vi "Write DAQ Rack Data.vi"(8 "Cal Unit":T2, 9 "Channel to Cal":T1, 10 "Verify Table":string[][](array[string]), 11 "Cal Path":path) -> ()   [LabVIEW 2013]
uses:
  Type Defs/Units Type Def (DAQ Rack).ctl
  Type Defs/Channel Type Def (RIO).ctl
  Type Defs/Excel Driver Operator Type Def.ctl
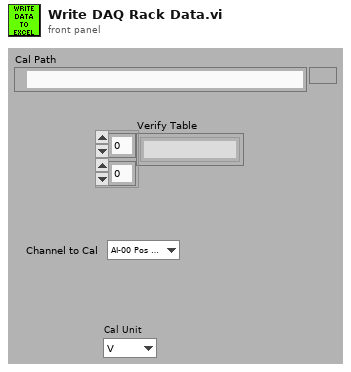
[diagram p1: front panel]
types:
  T1 = typedef "Channel Type Def (RIO).ctl" = enum16{"AI-00 Pos 1 Pump Current", "AI-01 Pos 2 Pump Current", "AI-02 Pos 3 Pump Current", "AI-03 Pos 4 Pump Current", "AI-04 Pos 5 Pump Current", "AI-05 Pos 6 Pump Current", "AI-06 Pos 1 Speed", "AI-07 Pos 2 speed", "AI-08 Pos 3 Speed", "AI-09 Pos 4 Speed", "AI-10 Pos 5 Speed", "AI-11 Pos 6 Speed", "AI-12 Pos 1 Controller Current", "AI-13 Pos 2 Controller Current", "AI-14 Pos 3 Controller Current", "AI-15 Pos 4 Controller Current", "AI-16 Pos 5 Controller Current", "AI-17 Pos 6 Controller Current", "AI-18 Spare", "AI-19 Tank 1 Temperature", "AI-20 Tank 2 Temperature", "AI-21 Power Supply Voltage", "AI-22 Pos 1 Pressure", "AI-23 Pos 2 Pressure", "AI-24 Pos 3 Pressure", "AI-25 Pos 4 Pressure", "AI-26 Pos 5 Pressure", "AI-27 Pos 6 Pressure", "AI-28 Pos 1 Flow", "AI-29 Pos 2 Flow", "AI-30 Pos 3 Flow", "AI-31 Pos 4 Flow", "AI-32 Pos 5 Flow", "AI-33 Pos 6 Flow", "AI-34 Spare", "AI-35 Spare", "AI-36 Spare", "AI-37 Spare"}
  T2 = typedef "Units Type Def (DAQ Rack).ctl" = enum16{"V", "mA", "A", "Hz", "deg C"}
  T3 = typedef "Excel Driver Operator Type Def.ctl" = enum16{"Open", "Close", "Search for String", "GetUsedRange", "Read Range", "Read Cell", "Set Range", "Set Cell"}
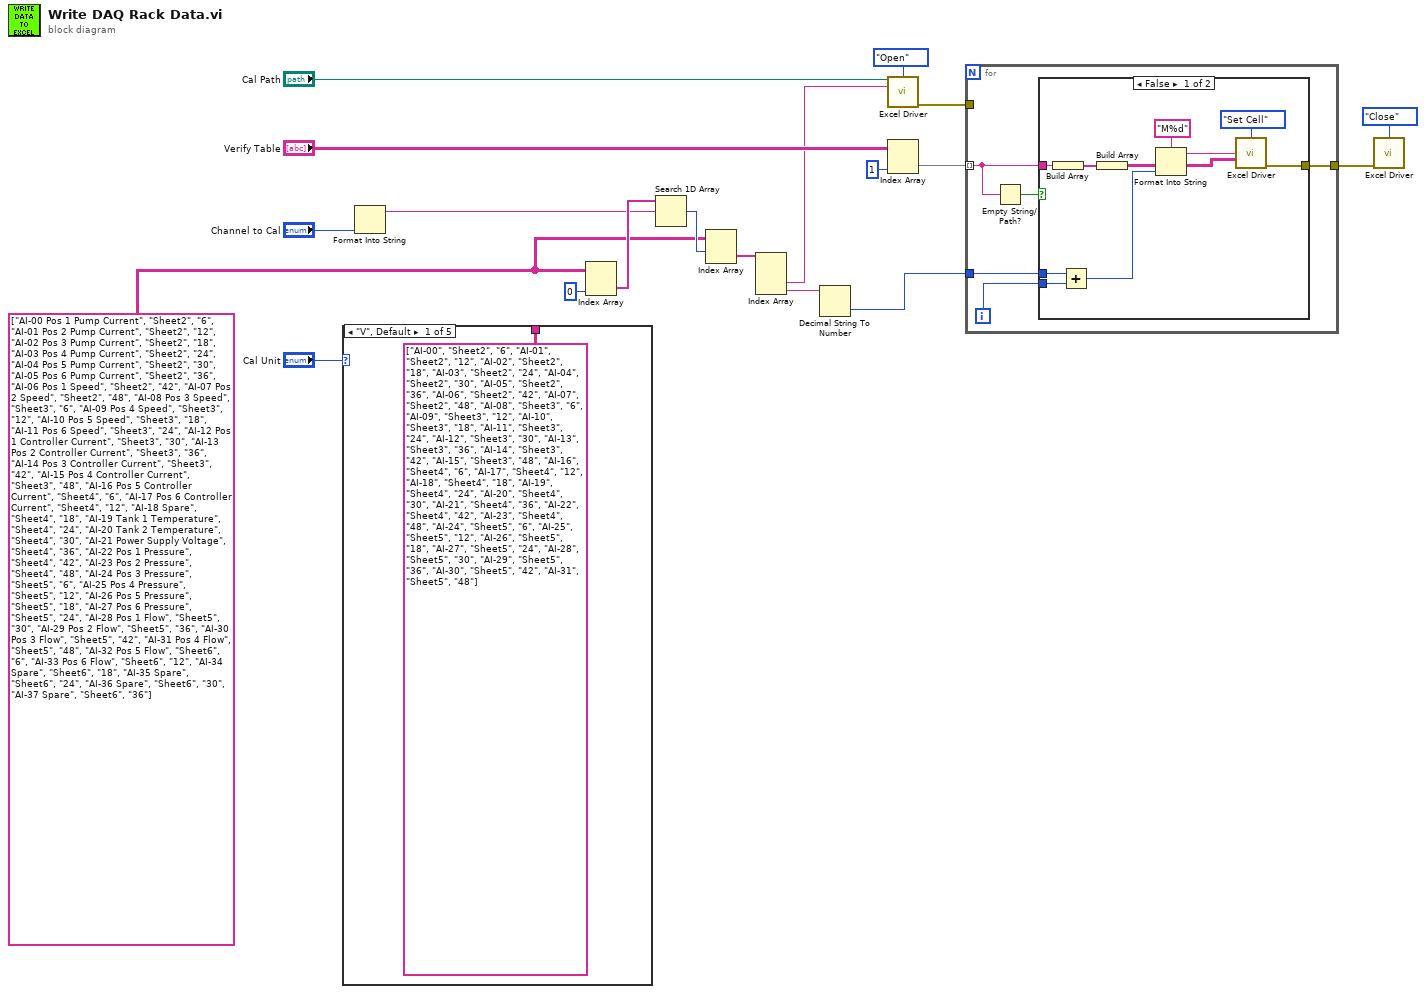
[diagram p0: block diagram]
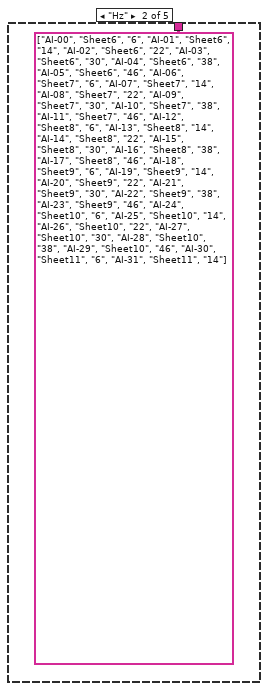
[diagram p2: hidden frame]
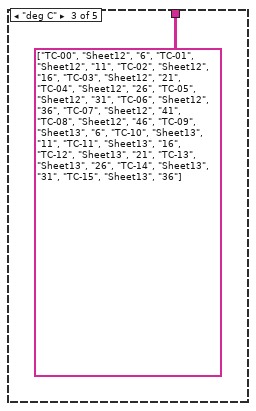
[diagram p3: hidden frame]
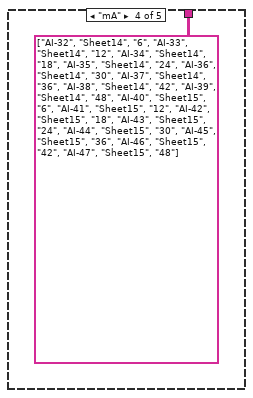
[diagram p4: hidden frame]
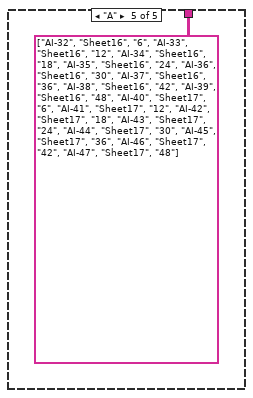
[diagram p5: hidden frame]
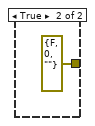
[diagram p6: hidden frame]
diagram:
  w1 = string[][] [["AI-00 Pos 1 Pump Current", "Sheet2", "6"], ["AI-01 Pos 2 Pump Current", "Sheet2", "12"], ["AI-02 Pos 3 Pump Current", "Sheet2", "18"], ["AI-03 Pos 4 Pump Current", "Sheet2", "24"], ["AI-04 Pos 5 Pump Current", "Sheet2", "30"], ["AI-05 Pos 6 Pump Current", "Sheet2", "36"], ["AI-06 Pos 1 Speed", "Sheet2", "42"], ["AI-07 Pos 2 Speed", "Sheet2", "48"], ["AI-08 Pos 3 Speed", "Sheet3", "6"], ["AI-09 Pos 4 Speed", "Sheet3", "12"], ["AI-10 Pos 5 Speed", "Sheet3", "18"], ["AI-11 Pos 6 Speed", "Sheet3", "24"], ["AI-12 Pos 1 Controller Current", "Sheet3", "30"], ["AI-13 Pos 2 Controller Current", "Sheet3", "36"], ["AI-14 Pos 3 Controller Current", "Sheet3", "42"], ["AI-15 Pos 4 Controller Current", "Sheet3", "48"], ["AI-16 Pos 5 Controller Current", "Sheet4", "6"], ["AI-17 Pos 6 Controller Current", "Sheet4", "12"], ["AI-18 Spare", "Sheet4", "18"], ["AI-19 Tank 1 Temperature", "Sheet4", "24"], ["AI-20 Tank 2 Temperature", "Sheet4", "30"], ["AI-21 Power Supply Voltage", "Sheet4", "36"], ["AI-22 Pos 1 Pressure", "Sheet4", "42"], ["AI-23 Pos 2 Pressure", "Sheet4", "48"], ["AI-24 Pos 3 Pressure", "Sheet5", "6"], ["AI-25 Pos 4 Pressure", "Sheet5", "12"], ["AI-26 Pos 5 Pressure", "Sheet5", "18"], ["AI-27 Pos 6 Pressure", "Sheet5", "24"], ["AI-28 Pos 1 Flow", "Sheet5", "30"], ["AI-29 Pos 2 Flow", "Sheet5", "36"], ["AI-30 Pos 3 Flow", "Sheet5", "42"], ["AI-31 Pos 4 Flow", "Sheet5", "48"], ["AI-32 Pos 5 Flow", "Sheet6", "6"], ["AI-33 Pos 6 Flow", "Sheet6", "12"], ["AI-34 Spare", "Sheet6", "18"], ["AI-35 Spare", "Sheet6", "24"], ["AI-36 Spare", "Sheet6", "30"], ["AI-37 Spare", "Sheet6", "36"]] ("deleted portion")
  n1 = case shown="\"V\", Default" "Cal Unit" {
    tunnel: [string[][] [["AI-00", "Sheet2", "6"], ["AI-01", "Sheet2", "12"], ["AI-02", "Sheet2", "18"], ["AI-03", "Sheet2", "24"], ["AI-04", "Sheet2", "30"], ["AI-05", "Sheet2", "36"], ["AI-06", "Sheet2", "42"], ["AI-07", "Sheet2", "48"], ["AI-08", "Sheet3", "6"], ["AI-09", "Sheet3", "12"], ["AI-10", "Sheet3", "18"], ["AI-11", "Sheet3", "24"], ["AI-12", "Sheet3", "30"], ["AI-13", "Sheet3", "36"], ["AI-14", "Sheet3", "42"], ["AI-15", "Sheet3", "48"], ["AI-16", "Sheet4", "6"], ["AI-17", "Sheet4", "12"], ["AI-18", "Sheet4", "18"], ["AI-19", "Sheet4", "24"], ["AI-20", "Sheet4", "30"], ["AI-21", "Sheet4", "36"], ["AI-22", "Sheet4", "42"], ["AI-23", "Sheet4", "48"], ["AI-24", "Sheet5", "6"], ["AI-25", "Sheet5", "12"], ["AI-26", "Sheet5", "18"], ["AI-27", "Sheet5", "24"], ["AI-28", "Sheet5", "30"], ["AI-29", "Sheet5", "36"], ["AI-30", "Sheet5", "42"], ["AI-31", "Sheet5", "48"]] ("deleted portion") string[][] [["AI-00", "Sheet6", "6"], ["AI-01", "Sheet6", "14"], ["AI-02", "Sheet6", "22"], ["AI-03", "Sheet6", "30"], ["AI-04", "Sheet6", "38"], ["AI-05", "Sheet6", "46"], ["AI-06", "Sheet7", "6"], ["AI-07", "Sheet7", "14"], ["AI-08", "Sheet7", "22"], ["AI-09", "Sheet7", "30"], ["AI-10", "Sheet7", "38"], ["AI-11", "Sheet7", "46"], ["AI-12", "Sheet8", "6"], ["AI-13", "Sheet8", "14"], ["AI-14", "Sheet8", "22"], ["AI-15", "Sheet8", "30"], ["AI-16", "Sheet8", "38"], ["AI-17", "Sheet8", "46"], ["AI-18", "Sheet9", "6"], ["AI-19", "Sheet9", "14"], ["AI-20", "Sheet9", "22"], ["AI-21", "Sheet9", "30"], ["AI-22", "Sheet9", "38"], ["AI-23", "Sheet9", "46"], ["AI-24", "Sheet10", "6"], ["AI-25", "Sheet10", "14"], ["AI-26", "Sheet10", "22"], ["AI-27", "Sheet10", "30"], ["AI-28", "Sheet10", "38"], ["AI-29", "Sheet10", "46"], ["AI-30", "Sheet11", "6"], ["AI-31", "Sheet11", "14"]] ("deleted portion") string[][] [["TC-00", "Sheet12", "6"], ["TC-01", "Sheet12", "11"], ["TC-02", "Sheet12", "16"], ["TC-03", "Sheet12", "21"], ["TC-04", "Sheet12", "26"], ["TC-05", "Sheet12", "31"], ["TC-06", "Sheet12", "36"], ["TC-07", "Sheet12", "41"], ["TC-08", "Sheet12", "46"], ["TC-09", "Sheet13", "6"], ["TC-10", "Sheet13", "11"], ["TC-11", "Sheet13", "16"], ["TC-12", "Sheet13", "21"], ["TC-13", "Sheet13", "26"], ["TC-14", "Sheet13", "31"], ["TC-15", "Sheet13", "36"]] ("array w/ subset deleted") string[][] [["AI-32", "Sheet14", "6"], ["AI-33", "Sheet14", "12"], ["AI-34", "Sheet14", "18"], ["AI-35", "Sheet14", "24"], ["AI-36", "Sheet14", "30"], ["AI-37", "Sheet14", "36"], ["AI-38", "Sheet14", "42"], ["AI-39", "Sheet14", "48"], ["AI-40", "Sheet15", "6"], ["AI-41", "Sheet15", "12"], ["AI-42", "Sheet15", "18"], ["AI-43", "Sheet15", "24"], ["AI-44", "Sheet15", "30"], ["AI-45", "Sheet15", "36"], ["AI-46", "Sheet15", "42"], ["AI-47", "Sheet15", "48"]] ("deleted portion") string[][] [["AI-32", "Sheet16", "6"], ["AI-33", "Sheet16", "12"], ["AI-34", "Sheet16", "18"], ["AI-35", "Sheet16", "24"], ["AI-36", "Sheet16", "30"], ["AI-37", "Sheet16", "36"], ["AI-38", "Sheet16", "42"], ["AI-39", "Sheet16", "48"], ["AI-40", "Sheet17", "6"], ["AI-41", "Sheet17", "12"], ["AI-42", "Sheet17", "18"], ["AI-43", "Sheet17", "24"], ["AI-44", "Sheet17", "30"], ["AI-45", "Sheet17", "36"], ["AI-46", "Sheet17", "42"], ["AI-47", "Sheet17", "48"]] ("deleted portion")] -> _
    frame "V", Default {
    }
    frame "Hz" {
    }
    frame "deg C" {
    }
    frame "mA" {
    }
    frame "A" {
    }
  }
  n2 = Format Into String("Channel to Cal") -> (resulting string=w3:string)  [unwired: 3 in, 1 out]
  n3 = Index Array(array=w1, index (col)=0 ("disabled index (col)")) -> (element=w10:string[])  [unwired: 1 in]
  n4 = Search 1D Array(1D array=w10, element=w3) -> (index of element=w9:i32)  [unwired: 1 in]
  n5 = Index Array(array=w1, index (row)=w9) -> (element=w8:string[])  [unwired: 1 in]
  n6 = Index Array(array=w8) -> (element #2=w7:string, element #3=w6:string)  [unwired: 3 in, 1 out]
  n7 = Decimal String To Number(string=w6) -> (number=w5:i32)  [unwired: 2 in, 1 out]
  n8 = call "Excel Driver.vi"("Filename of Workbook"="Cal Path", "Operator"=Excel_Driver_Operator_Type_Def."Open", "WorkSheet Name"=w7) -> ("error out"=w15:errorcluster)  [unwired: 10 in, 2 out]
  n9 = Index Array(array="Verify Table", index (col)=1 ("disabled index (col)")) -> (element=w16:string[])  [unwired: 1 in]
  n10 = for {
    tunnel: w16 -> [w26] mode=indexing
    tunnel: w5 -> [w29]
    tunnel: w15 -> [_]
    tunnel: [w28] -> w13
    i -> [w27]
    n11 = Empty String/Path?(string/path=w26) -> (empty?=w25:bool)
    n12 = case shown="False" w25 {
      tunnel: w26 -> [w38 _]
      tunnel: w29 -> [w32 _]
      tunnel: [w31 errorcluster {"status"=FALSE, "code"=0, "source"=""} ("error out")] -> w28
      tunnel: w27 -> [w30 _]
      frame False {
        n13 = Build Array(w38) -> (w37:string[])
        n14 = Add(x=w32, y=w30) -> (x+y=w33:i32)
        n15 = Build Array(w37) -> (w36:string[][])
        n16 = Format Into String(format string="M%d", w33) -> (resulting string=w34:string)  [unwired: 2 in, 1 out]
        n17 = call "Excel Driver.vi"("Operator"=Excel_Driver_Operator_Type_Def."Set Cell", "Range String\n(Or Search String)"=w34, "Cell Values INPUT"=w36) -> ("error out"=w31:errorcluster)  [unwired: 10 in, 2 out]
      }
      frame True {
      }
    }
  }
  n18 = call "Excel Driver.vi"("Operator"=Excel_Driver_Operator_Type_Def."Close", "error in (no error)"=w13) -> ()  [unwired: 11 in, 3 out]
